vi "Lab_3_START_Clusters_Files_SUBVI_Michal_Cedro.vi"(8 "Error IN":errorcluster, 11 "HR Data Structure IN":T1 {"Raw Data"."Time" format="%<%x %.3X>T"}) -> (0 "error out":errorcluster, 2 "Array":dbl[](array[numeric]), 3 "HR Data Structure OUT":T1 {"Raw Data"."Time" format="%<%x %.3X>T"})   [LabVIEW 2025]
uses:
  Controls/HR_Data_Structure.ctl
  Controls/Raw_Data_IN_HR.ctl
  Controls/Runner_Data_Structure.ctl
panel:
  out "FATIGUE":cluster{"Time":timestamp[], dbl[]}(graph)
  out "HEART RATE ZONE":string[][](array[string])
  out "XY Graph":cluster{dbl[], "Heart Rate Zone":i32[]}(graph)
  out "BPM":cluster{"Time":timestamp[], "Bpm":i32[]}(graph)
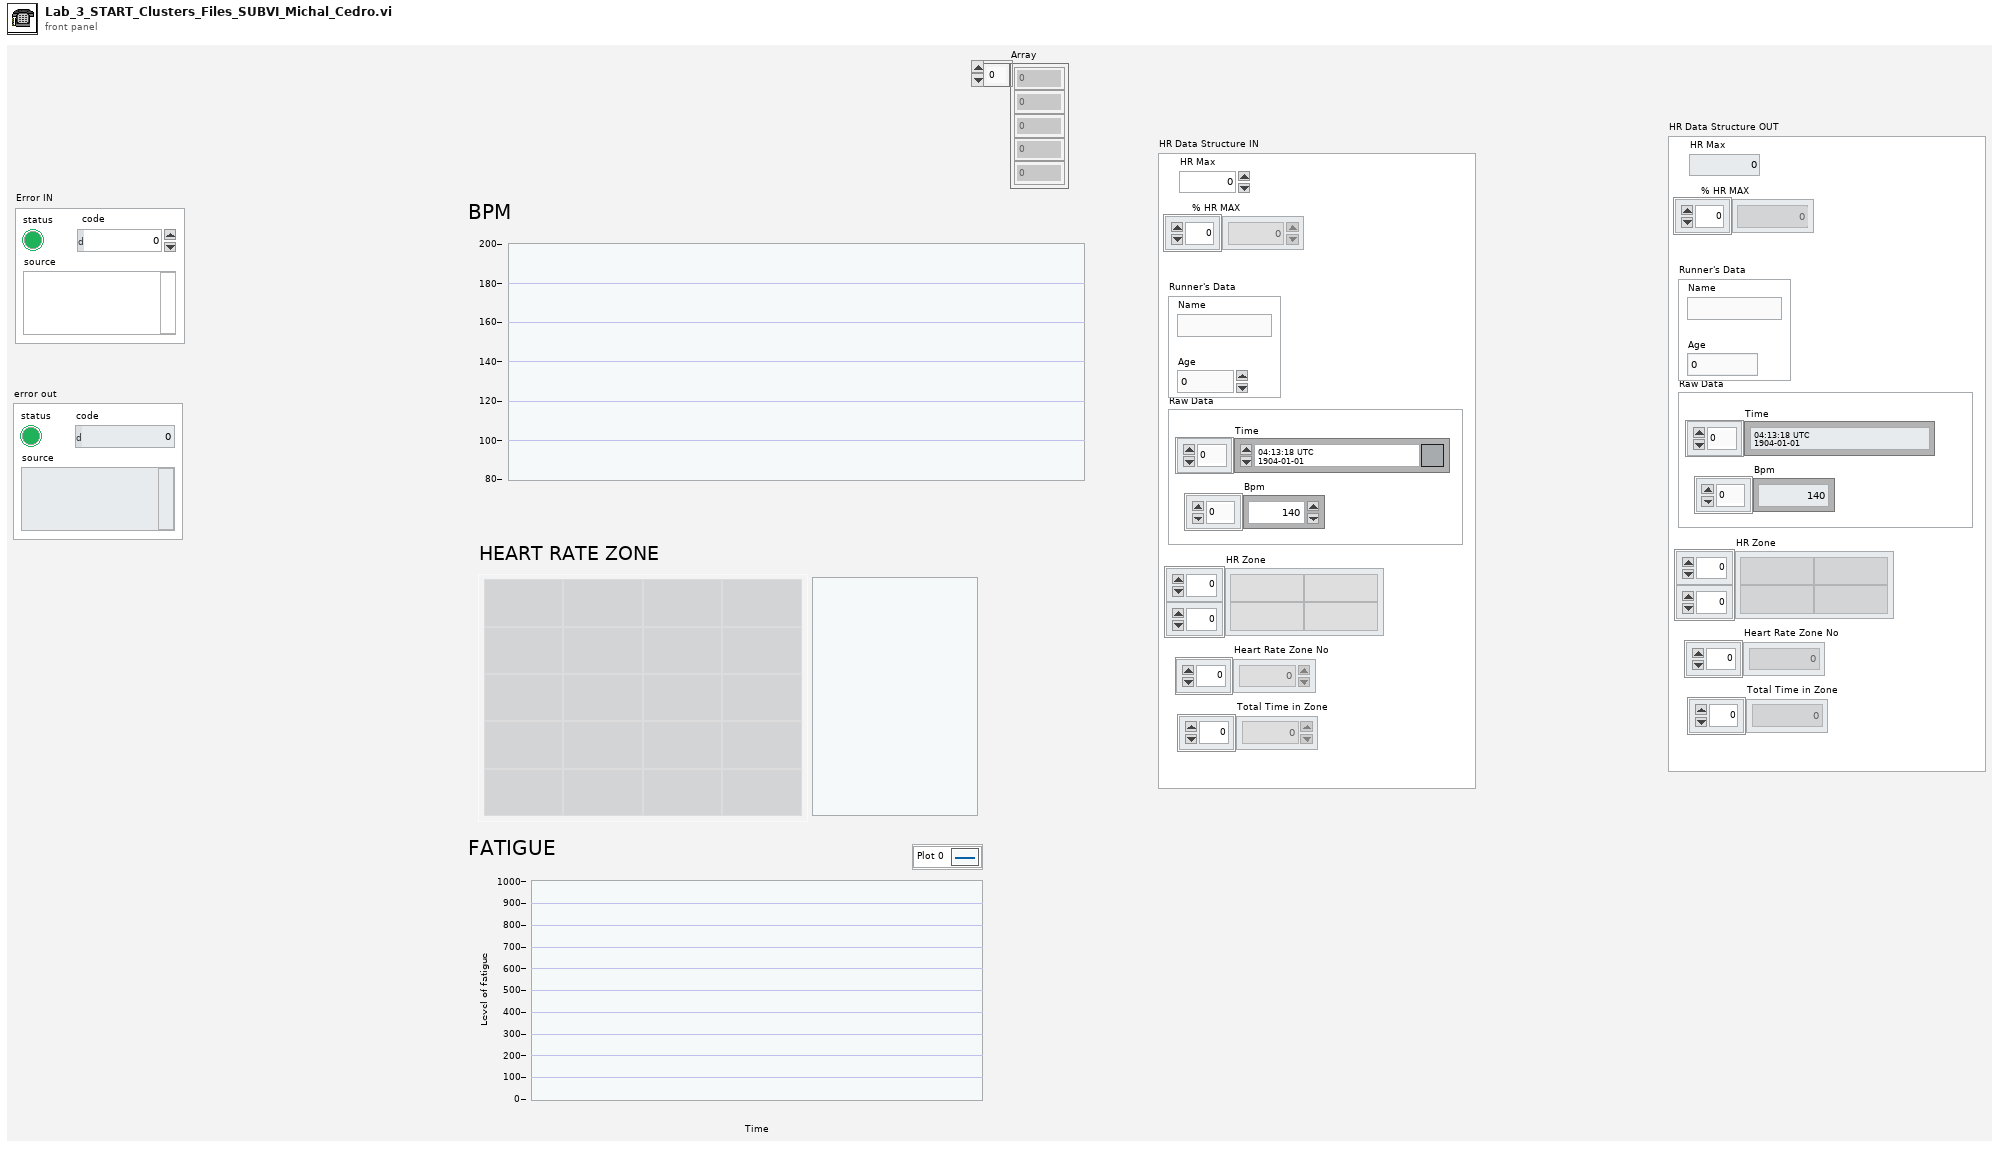
[diagram p1: front panel]
types:
  T1 = typedef "HR_Data_Structure.ctl" = cluster{"HR Max":i32, "% HR MAX ":dbl[], "Raw Data":T2, "Runner's Data":T3, "HR Zone":string[][], "Total Time in Zone":dbl[], "Heart Rate Zone No":dbl[]}
  T2 = typedef "Raw_Data_IN_HR.ctl" = cluster{"Time":timestamp[], "Bpm":i32[]}
  T3 = typedef "Runner_Data_Structure.ctl" = cluster{"Name":string, "Age":i32}
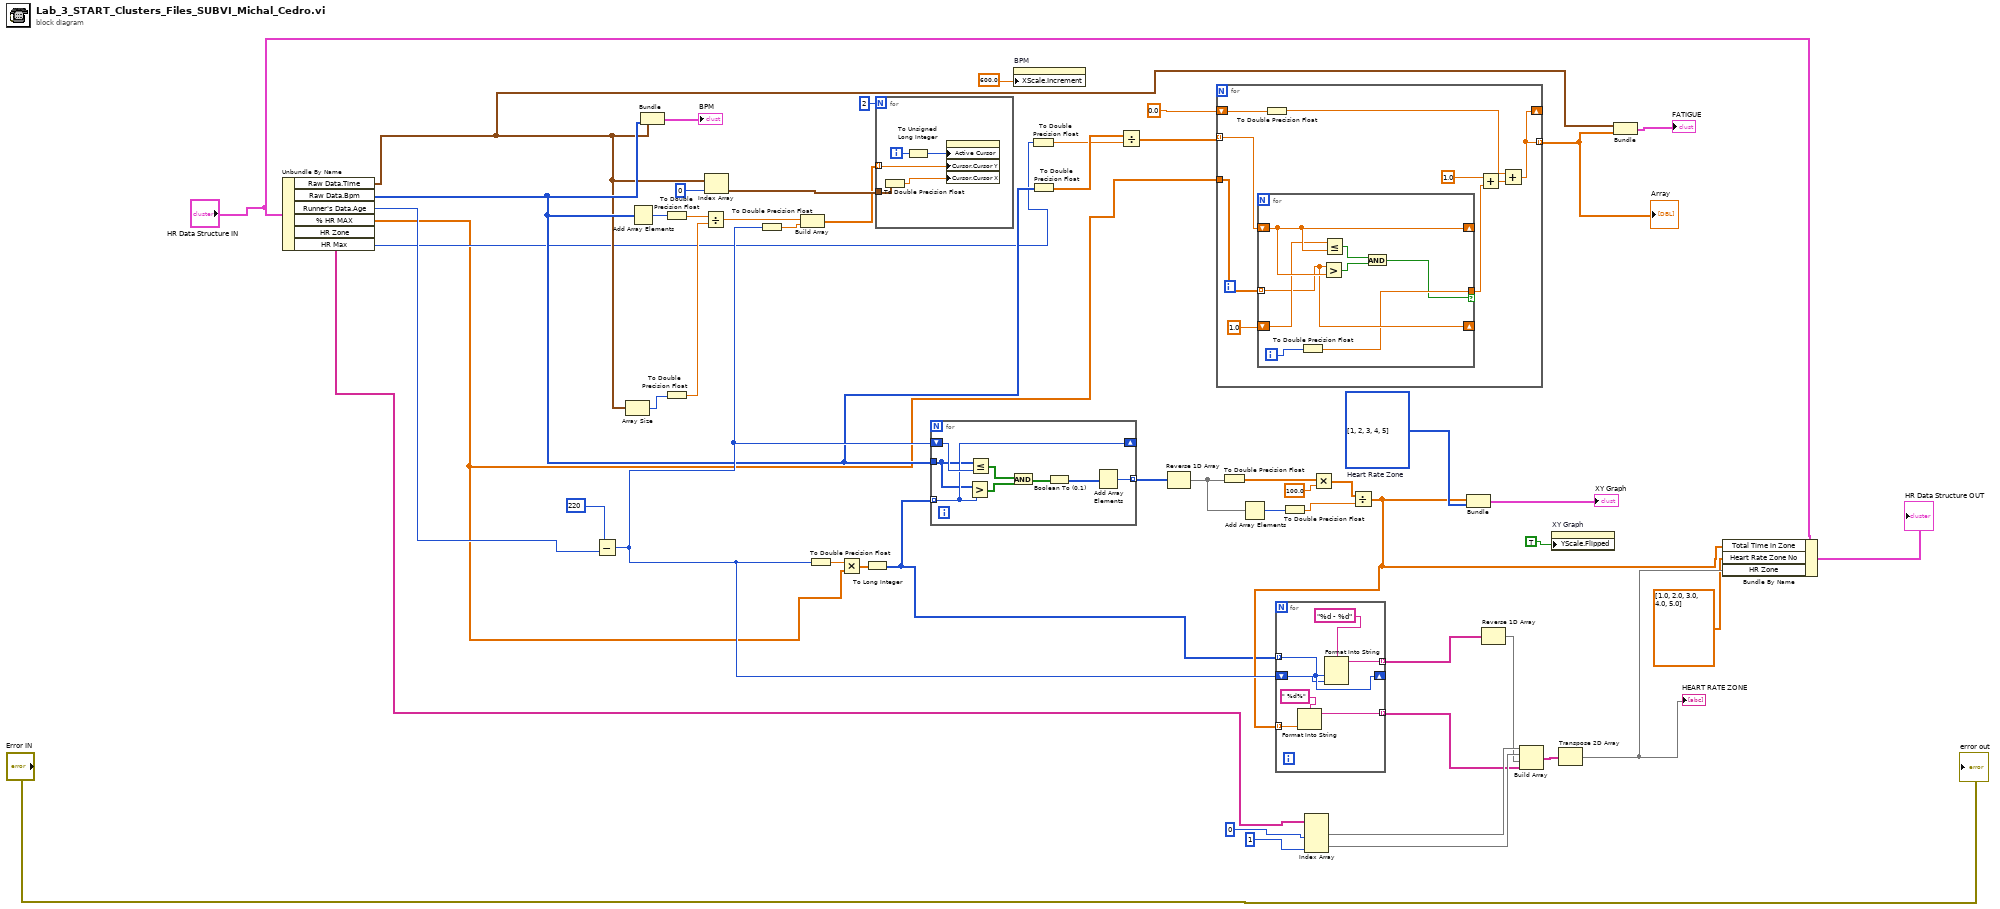
[diagram p0: block diagram]
diagram:
  w36 = i32[] [1, 2, 3, 4, 5]  # Heart Rate Zone
  n1 = Unbundle By Name("HR Data Structure IN") -> ("Raw Data.Time"=w7:timestamp[], "Raw Data.Bpm"=w11:i32[], "Runner's Data.Age"=w20:i32, "% HR MAX"=w1:dbl[], "HR Zone"=w19:string[][], "HR Max"=w3:i32)
  n2 = Subtract(x=220, y=w20) -> (x-y=w33:i32)
  n3 = Array Size(array=w7) -> (size(s)=w51:i32)
  n4 = Add Array Elements(numeric array=w11) -> (sum=w52:i32)
  n5 = Bundle("Time"=w7, "Bpm"=w11) -> (→"BPM":cluster{"Time":timestamp[], "Bpm":i32[]})  [unwired: 1 in]
  n6 = To Double Precision Float(number=w52) -> (double precision float=w50:dbl)
  n7 = To Double Precision Float(number=w51) -> (double precision float=w49:dbl)
  n8 = Divide(x=w50, y=w49) -> (x/y=w34:dbl)
  n9 = Index Array(array=w7, index=0) -> (element=w45:timestamp)
  n10 = To Double Precision Float(number=w33) -> (double precision float=w15:dbl)
  n11 = Build Array(w34, w15) -> (w32:dbl[])
  n12 = To Double Precision Float(number=w33) -> (double precision float=w48:dbl)
  n13 = Multiply(x=w48, y=w1) -> (x*y=w44:dbl[])
  n14 = To Long Integer(number=w44) -> (32bit integer=w4:i32[])
  n15 = for {
    N: 2 -> [_]
    tunnel: w32 -> [w56] mode=indexing
    tunnel: w45 -> [w58]
    i -> [w55]
    n16 = To Double Precision Float(number=w58) -> (double precision float=w57:dbl)
    n17 = To Unsigned Long Integer(number=w55) -> (unsigned 32bit integer=w54:u32)
    n18 = property on="BPM" class="XYGraph (strict)"("Active Cursor"=w54, "Cursor.Cursor Y"=w56, "Cursor.Cursor X"=w57) -> ()  [unwired: 2 in, 2 out]
  }
  n19 = for {
    tunnel: w4 -> [w60] mode=indexing
    tunnel: w11 -> [w59]
    shift-right: [w60] -> _
    shift-left: w33 -> [w66]
    tunnel: [w65] -> w43 mode=indexing
    n20 = Greater?(x=w59, y=w60) -> (0:w62:bool[])
    n21 = Less Or Equal?(x=w59, y=w66) -> (x <= y?=w63:bool[])
    n22 = And(x=w63, y=w62) -> (x .and. y?=w61:bool[])
    n23 = Boolean To (0,1)(Boolean=w61) -> (0, 1=w64:i16[])
    n24 = Add Array Elements(numeric array=w64) -> (sum=w65:i16)
  }
  n25 = property on="BPM" class="XYGraph (strict)"("XScale.Increment"=600.0) -> ()  [unwired: 2 in, 2 out]
  n26 = To Double Precision Float(number=w3) -> (double precision float=w2:dbl)
  n27 = To Double Precision Float(number=w11) -> (double precision float=w10:dbl[])
  n28 = Divide(x=w10, y=w2) -> (x/y=w9:dbl[])
  n29 = Reverse 1D Array(array=w43) -> (reversed array=w42:i16[])
  n30 = for {
    tunnel: w1 -> [w70]
    tunnel: w9 -> [w69] mode=indexing
    shift-right: [w71] -> _
    shift-left: 0.0 -> [w73]
    tunnel: [w71] -> w5 mode=indexing
    n31 = for {
      tunnel: w70 -> [w79] mode=indexing
      shift-right: [w81] -> _
      shift-left: w69 -> [w81]
      shift-right: [w79] -> _
      shift-left: 1.0 -> [w80]
      tunnel: [w77] -> w67 if=w76
      i -> [w78]
      n32 = To Double Precision Float(number=w78) -> (double precision float=w77:dbl)
      n33 = Greater?(x=w79, y=w81) -> (0:w82:bool)
      n34 = Less Or Equal?(x=w80, y=w81) -> (x <= y?=w83:bool)
      n35 = And(x=w83, y=w82) -> (x .and. y?=w76:bool)
    }
    n36 = To Double Precision Float(number=w73) -> (double precision float=w72:dbl)
    n37 = Add(x=1.0, y=w67) -> (x+y=w74:dbl)
    n38 = Add(x=w72, y=w74) -> (x+y=w71:dbl)
  }
  "Array" <- w5
  n39 = To Double Precision Float(number=w42) -> (double precision float=w41:dbl[])
  n40 = Add Array Elements(numeric array=w42) -> (sum=w39:i16)
  n41 = To Double Precision Float(number=w39) -> (double precision float=w37:dbl)
  n42 = Index Array(array=w19, index (col) #1=0, index (col) #2=1) -> (element #1=w29:string[], element #2=w28:string[])  [unwired: 2 in]
  n43 = Multiply(x=w41, y=100.0) -> (x*y=w38:dbl[])
  n44 = Divide(x=w38, y=w37) -> (x/y=w13:dbl[])
  n45 = for {
    tunnel: w4 -> [w89] mode=indexing
    tunnel: [w90] -> w35 mode=indexing
    shift-right: [w89] -> _
    shift-left: w33 -> [w88]
    tunnel: w13 -> [w87] mode=indexing
    tunnel: [w86] -> w26 mode=indexing
    n46 = Format Into String(format string=" %d%", w87) -> (resulting string=w86:string)  [unwired: 2 in, 1 out]
    n47 = Format Into String(format string="%d - %d", w89, w88) -> (resulting string=w90:string)  [unwired: 2 in, 1 out]
  }
  n48 = Bundle(w13, "Heart Rate Zone"=w36) -> (→"XY Graph":cluster{dbl[], "Heart Rate Zone":i32[]})  [unwired: 1 in]
  n49 = Reverse 1D Array(array=w35) -> (reversed array=w27:string[])
  n50 = Build Array(w29, w28, w27, w26) -> (w25:string[][])
  n51 = property on="XY Graph" class="XYGraph (strict)"("YScale.Flipped"=TRUE) -> ()  [unwired: 2 in, 2 out]
  n52 = Transpose 2D Array(2D array=w25) -> (transposed array=w16:string[][])
  "HEART RATE ZONE" <- w16
  n53 = Bundle("Time"=w7, w5) -> (→"FATIGUE":cluster{"Time":timestamp[], dbl[]})  [unwired: 1 in]
  n54 = Bundle By Name(cluster="HR Data Structure IN", "Total Time in Zone"=w13, "Heart Rate Zone No"=dbl[] [1.0, 2.0, 3.0, 4.0, 5.0], "HR Zone"=w16) -> (→"HR Data Structure OUT":T1)
  "error out" <- "Error IN"
